vi "Interrupt.vi"(11 "Enum":T3) -> (0 "Voltage":dbl, 3 "InterruptRef":T1={"DevStatus"={"status"=FALSE, "code"=0, "source"=""}, "InterruptIndex"=enum."Invalid"})   [LabVIEW 2014]
uses:
  TypeDefs/SRE Enum.ctl
  <vilib>/Rock Robotics/WPI/Interrupt/WPI_InterruptRef.ctl
  <vilib>/Rock Robotics/SystemInterfaces/Interrupt/FPGA_InterruptIndex.ctl
  <vilib>/Rock Robotics/SystemInterfaces/AI/FPGA_AIChannel.ctl
  <vilib>/Rock Robotics/WPI/Counter/WPI_CounterAnalogTriggerToDigitalSource.vi
  <vilib>/Rock Robotics/SystemInterfaces/CounterEncoderSourceConvertion/FPGA_CounterEncoderSourceConvertionLVSourceTypeToFPGAType.vi
  <vilib>/Rock Robotics/WPI/Interrupt/WPI_InterruptCache.vi
  <vilib>/Rock Robotics/SystemInterfaces/Interrupt/FPGA_InterruptWriteConfiguration.vi
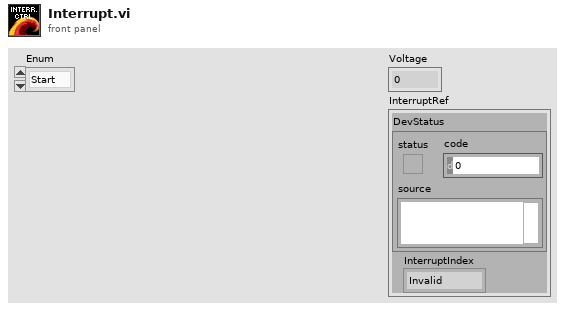
[diagram p1: front panel]
types:
  T1 = typedef "WPI_InterruptRef.ctl" = cluster{"DevStatus":errorcluster, "InterruptIndex":T2}
  T2 = typedef "FPGA_InterruptIndex.ctl" = enum8{"0", "1", "2", "3", "4", "5", "6", "7", "Invalid"}
  T3 = typedef "SRE Enum.ctl" = enum16{"Start", "Run", "End"}
  T4 = typedef "FPGA_AIChannel.ctl" = enum8{"AI 0", "AI 1", "AI 2", "AI 3", "AI MXP 0", "AI MXP 1", "AI MXP 2", "AI MXP 3", "Invalid"}
  T5 = typedef "WPI_AnalogChannelDevRef.ctl" = cluster{"DevStatus":errorcluster, "Controller":T6, "Analog Channel":T4}
  T6 = typedef "FPGA_TypedefAnalogModule.ctl" = enum16{"Controller 1"}
  T7 = typedef "FPGA_AnalogTriggerDevRef.ctl" = cluster{"DevStatus":errorcluster, "AnalogTriggerIndex":T8}
  T8 = typedef "FPGA_AnalogTriggerIndex.ctl" = enum8{"Trig 0", "Trig 1", "Trig 2", "Trig 3", "Trig 4", "Trig 5", "Trig 6", "Trig 7", "Invalid"}
  T9 = typedef "FPGA_CounterEncoderSourceConvertionLVSourceType.ctl" = cluster{"DevStatus":errorcluster, "AnalogTriggerMode?":bool, "DigitalMode":cluster{"Controller":T10, "DIO Channel":T11}, "AnalogTriggerMode":cluster{"AnalogTriggerIndex":T8, "OutputType":T12}}
  T10 = typedef "FPGA_TypedefDigitalModule.ctl" = enum16{"Controller 1"}
  T11 = typedef "FPGA_DIODigitalSourceChannel.ctl" = enum8{"DIO 0", "DIO 1", "DIO 2", "DIO 3", "DIO 4", "DIO 5", "DIO 6", "DIO 7", "DIO 8", "DIO 9", "DIO MXP 0", "DIO MXP 1", "DIO MXP 2", "DIO MXP 3", "DIO MXP 4", "DIO MXP 5", "DIO MXP 6", "DIO MXP 7", "DIO MXP 8", "DIO MXP 9", "DIO MXP 10", "DIO MXP 11", "DIO MXP 12", "DIO MXP 13", "DIO MXP 14", "DIO MXP 15", "Disabled"}
  T12 = typedef "FPGA_AnalogTriggerOutType.ctl" = enum16{"InWindow", "TriggerState", "Rising", "Falling"}
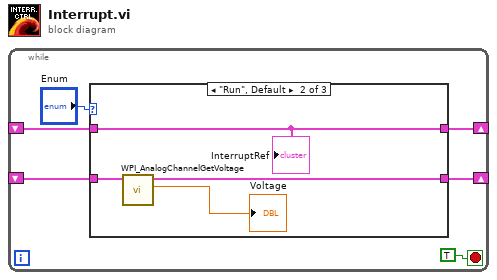
[diagram p0: block diagram]
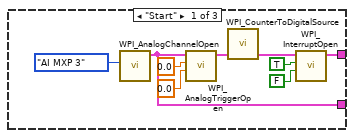
[diagram p2: hidden frame]
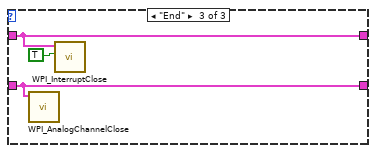
[diagram p3: hidden frame]
diagram:
  n1 = while {
    shift-right: [w4] -> _
    shift-left: _ -> [w5]
    shift-right: [w1] -> _
    shift-left: _ -> [w2]
    stop <- TRUE stop-if-true
    n2 = case shown="\"Run\", Default" "Enum" {
      tunnel: w5 -> [_ w16 w22]
      tunnel: [w15 w16 w22] -> w4
      tunnel: [w9 w18 w20] -> w1
      tunnel: w2 -> [_ w19 w20]
      frame "Start" {
        n3 = call <vilib>:"WPI_AnalogChannelOpen.vi"("Analog Channel"=FPGA_AIChannel."AI MXP 3") -> ("AIDeviceRef"=w9:T5)  [unwired: 9 in, 1 out]
        n4 = call <vilib>:"WPI_AnalogTriggerOpen.vi"("LowerLimit (v)"=0.0, "UpperLimit (v)"=0.0, "AnalogTriggerSource"=w9) -> ("AnalogTriggerDevRef"=w13:T7)  [unwired: 7 in, 1 out]
        n5 = call-poly <vilib>:"WPI_CounterToDigitalSource.vi"("AnalogTriggerDevRef"=w13) -> ("Digital Source"=w14:T9)  [unwired: 6 in]
        n6 = call <vilib>:"WPI_InterruptOpen.vi"("Falling Edge"=FALSE, "Rising Edge"=TRUE, "Source"=w14) -> ("InterruptRef"=w15:T1)  [unwired: 7 in, 1 out]
      }
      frame "Run", Default {
        n7 = call <vilib>:"WPI_AnalogChannelGetVoltage.vi"("AIDeviceRef"=w19) -> ("Voltage"=→"Voltage":dbl, "AIDeviceRef"=w18:T5)  [unwired: 8 in, 1 out]
        "InterruptRef" <- w16
      }
      frame "End" {
        n8 = call <vilib>:"WPI_AnalogChannelClose.vi"("AIDeviceRef"=w20) -> ()  [unwired: 10 in, 1 out]
        n9 = call <vilib>:"WPI_InterruptClose.vi"("Close Dependencies"=TRUE, "InterruptRef"=w22) -> ()  [unwired: 9 in, 1 out]
      }
    }
  }
